vi "Configure Alarm Hysteresis IO.vi"(0 "VISA resource name":refnum<visa-resource-name>, 5 "Channel (0001)":string="0001", 7 "Alarm No. (1)":i32=1 min=1 max=4, 9 "Measurement Channel Hysteresis (0)":i32 min=0 max=100000 step=1, 11 "error in (no error)":errorcluster) -> (4 "VISA resource name out":refnum<visa-resource-name>, 6 "Channel":string, 8 "Alarm No.":i32, 15 "error out":errorcluster)   [LabVIEW 2020, in "Yokogawa GX Series.lvlib"]
doc: "Sets the alarm hysteresis for the IO channel.\n\nCommand: SAlmHysIO"
uses:
  <instrlib>/Yokogawa GX Series/Yokogawa GX Series.lvlib
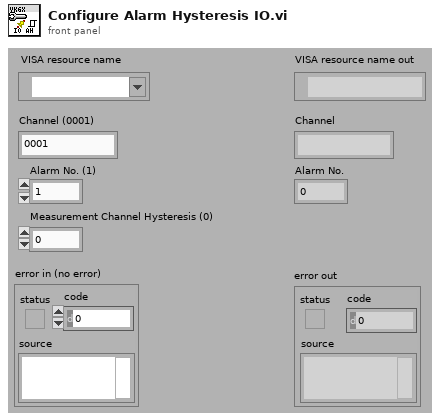
[diagram p1: front panel]
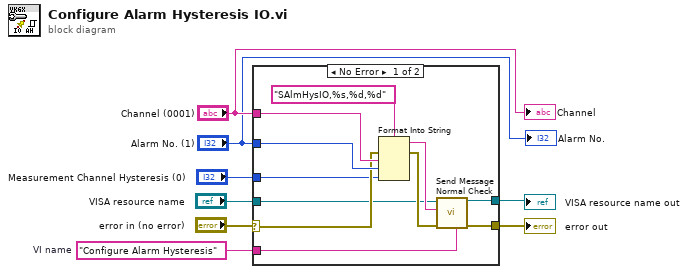
[diagram p0: block diagram]
diagram:
  w7 = "Configure Alarm Hysteresis"  # VI name
  n1 = case shown="No Error" "error in (no error)" {
    selector: "error in (no error)" -> [w11 w20]
    tunnel: "VISA resource name" -> [w10 w21]
    tunnel: w7 -> [w16 _]
    tunnel: [w15 w21] -> w6
    tunnel: [w14 w20] -> w5
    tunnel: "Measurement Channel Hysteresis (0)" -> [w9 _]
    tunnel: "Channel (0001)" -> [w13 _]
    tunnel: "Alarm No. (1)" -> [w12 _]
    frame No Error {
      n2 = Format Into String(format string="SAlmHysIO,%s,%d,%d", error in=w11, w13, w12, w9) -> (resulting string=w17:string, error out=w18:errorcluster)  [unwired: 1 in]
      n3 = call <instrlib>:"Send Message Normal Check.vi"("Source (\"\")"=w16, "error in (no error)"=w18, "Send Message (\"\")"=w17, "VISA resource name"=w10) -> ("error out"=w14:errorcluster, "VISA resource name out"=w15:refnum<visa-resource-name>)  [unwired: 2 in, 4 out]
    }
    frame Error {
    }
  }
  "error out" <- w5
  "VISA resource name out" <- w6
  "Channel" <- "Channel (0001)"
  "Alarm No." <- "Alarm No. (1)"
